vi "GT Get Follow Status.vi"(7 "pSwitchStatus":i16, 8 "error in (no error)":errorcluster caption="错误输入（无错误）", 9 "pFifoNum":i16, 10 "profile":i16, 11 "cardNum":i16) -> (0 "error out":errorcluster caption="错误输出", 1 "pFifoNum out":i16, 3 "function return":i16, 5 "pSwitchStatus out":i16)   [LabVIEW 2014, in "gts.lvlib"]
doc: "GT_API GT_GetFollowStatus(short cardNum,short profile,short *pFifoNum,short *pSwitchStatus);"
uses:
  gts.lvlib
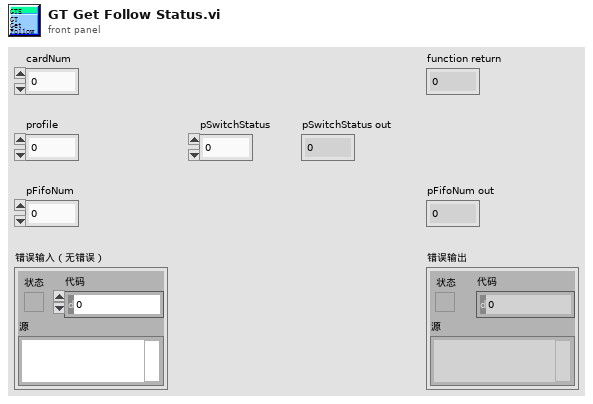
[diagram p1: front panel]
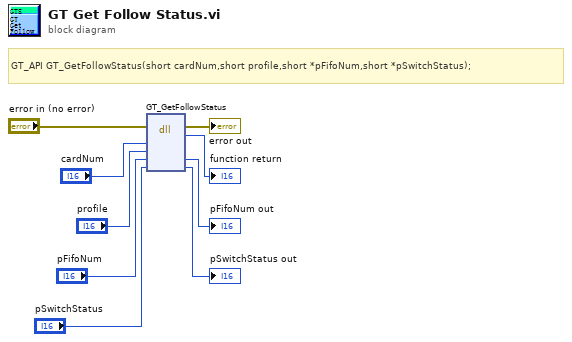
[diagram p0: block diagram]
diagram:
  # "GT_API GT_GetFollowStatus(short cardNum,short profile,short *pFifoNum,short *pSwitchStatus);"
  n1 = dll-call lib="PTH2habs D固高科技资料GTS控制卡GTS卡18年上半年资料dllVC32bit\nmulti_cardgts.*" fn="GT_GetFollowStatus"(error in="error in (no error)", "cardNum"="cardNum", "profile"="profile", "pFifoNum"="pFifoNum", "pSwitchStatus"="pSwitchStatus") -> (error out=→"error out":errorcluster, →"function return":i16, "pFifoNum"=→"pFifoNum out":i16, "pSwitchStatus"=→"pSwitchStatus out":i16)  [unwired: 4 in, 1 out]
